vi "探头窗口-20.vi"() -> ()   [LabVIEW 2017]
panel:
  in  "更新数据":T1
  in  "停止信号":bool=TRUE
  out "更新数据？":bool=TRUE
  out "引用-切回列表模式？":refnum<vi>
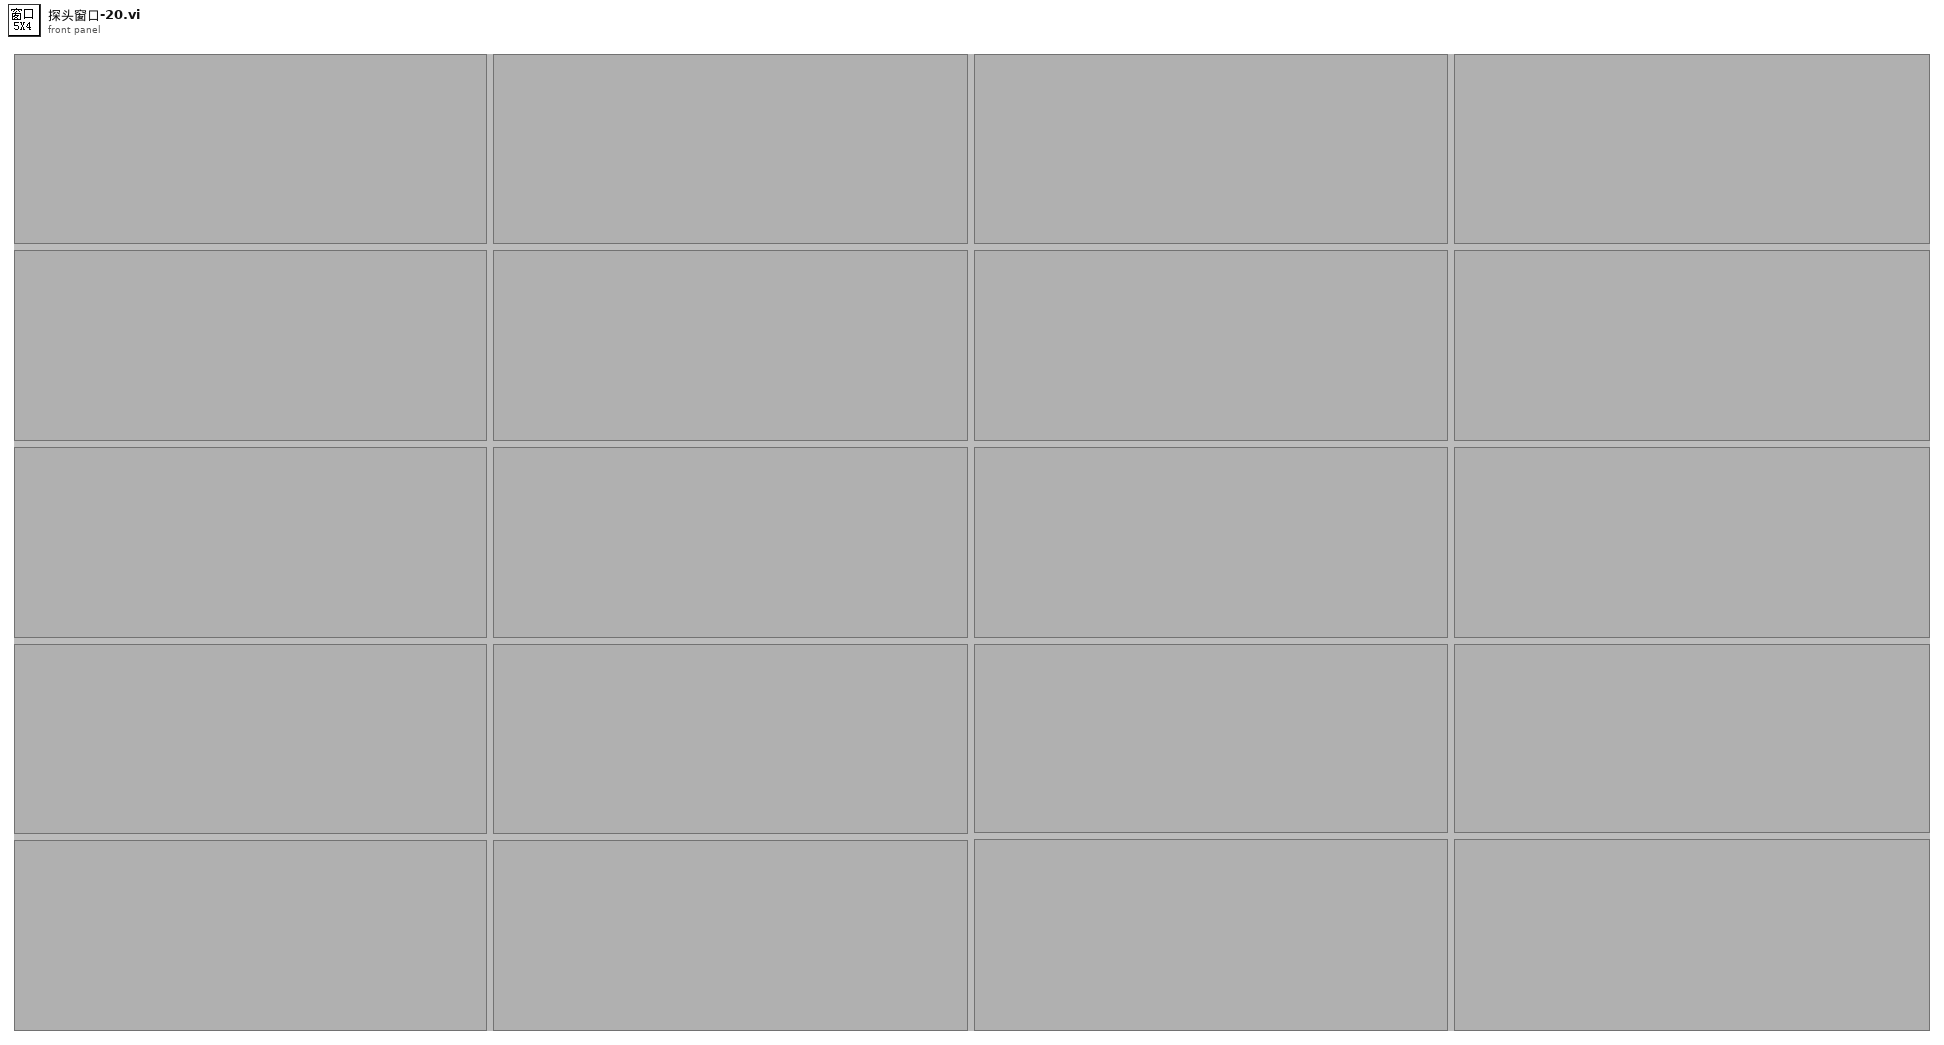
[diagram p1: front panel]
types:
  T1 = cluster{"探头启用状态？":bool[], "测量值":cluster{"X":timestamp, "Y":dbl}[], "限值":cluster{"限值1":dbl, "限值2":dbl, "探头限值":enum16{"一级限值", "二级限值"}}[], "报警状态":enum16{"正常", "一级报警", "二级报警", "累积报警"}[], "探头信息":string[], "累积剂量":cluster{"设备名称":string, "启用累积？":bool, "起始时间":timestamp, "累积剂量":dbl, "累积报警阈值":dbl}[]}
  T2 = cluster{"启用状态？":bool, "测量值":cluster{"X":timestamp, "Y":dbl}, "限值簇":cluster{"限值1":dbl, "限值2":dbl, "探头限值":enum16{"一级限值", "二级限值"}}, "报警状态":enum16{"正常", "一级报警", "二级报警", "累积报警"}, "探头信息":string, "探头地址":i32, "累积剂量":cluster{"设备名称":string, "启用累积？":bool, "起始时间":timestamp, "累积剂量":dbl, "累积报警阈值":dbl}}
  T3 = typedef "eventvkey.ctl" = enum16{"ASCII", "Enter", "Return", "Shift", "Ctrl", "Alt", "Cmd", "Opt", "Caps", "NumLock", "Clear", "Break", "Up", "Down", "Left", "Right", "Insert", "Delete", "Home", "End", "PageUp", "PageDown", "Escape", "Help", "Pause", "ScrollLock", "F1", "F2", "F3", "F4", "F5", "F6", "F7", "F8", "F9", "F10", "F11", "F12", "F13", "F14", "F15", "F16", "F17", "F18", "F19", "F20", "F21", "F22", "F23", "F24", "Play", "VolumeUp", "VolumeDown", "Mute", "Two Byte Char"}
  T4 = cluster{"限值1":dbl, "限值2":dbl, "探头限值":enum16{"一级限值", "二级限值"}}
  T5 = cluster{"限值1":dbl, "限值2":dbl, "探头限值":enum16{"一级限值", "二级限值"}}[]
  T6 = cluster{"设备名称":string, "启用累积？":bool, "起始时间":timestamp, "累积剂量":dbl, "累积报警阈值":dbl}[]
  T7 = cluster{"设备名称":string, "启用累积？":bool, "起始时间":timestamp, "累积剂量":dbl, "累积报警阈值":dbl}
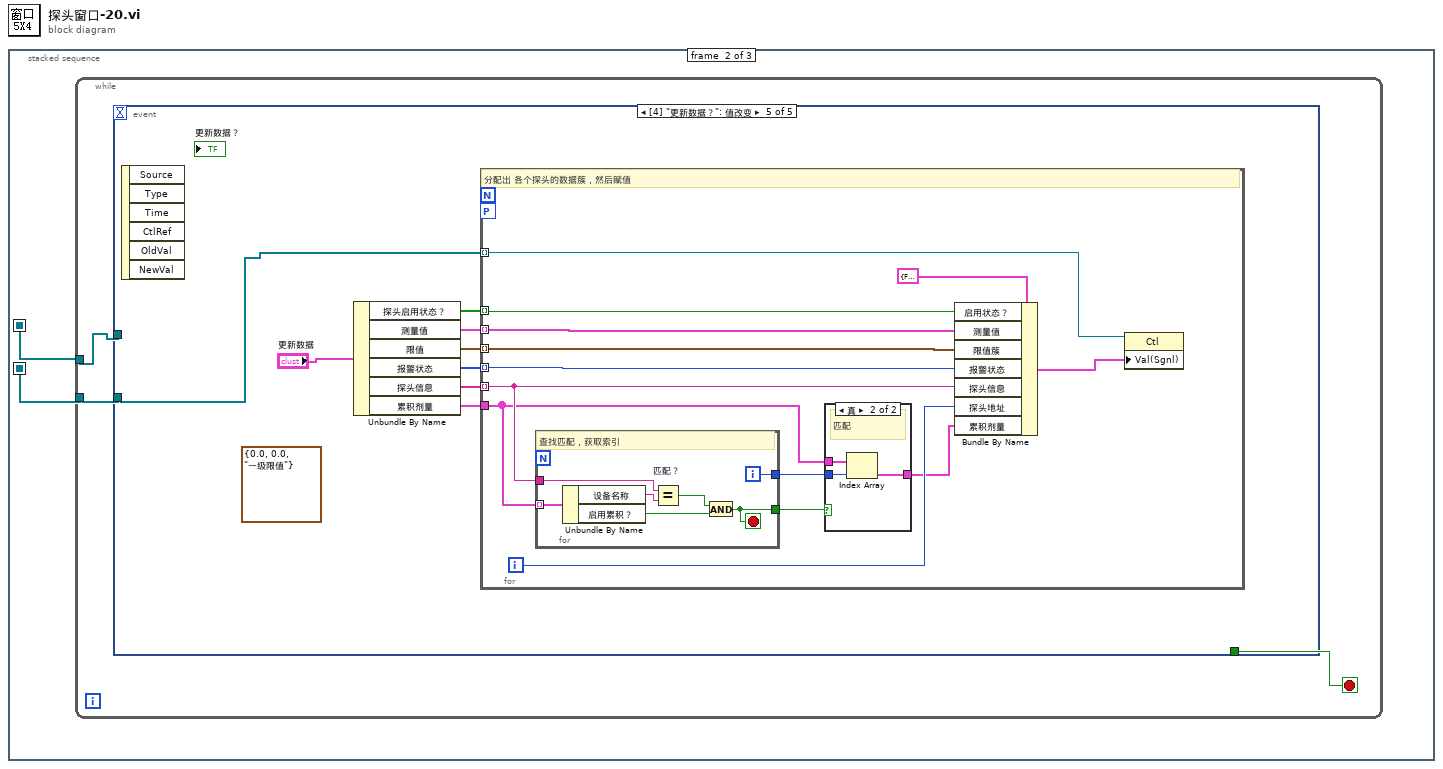
[diagram p0: block diagram]
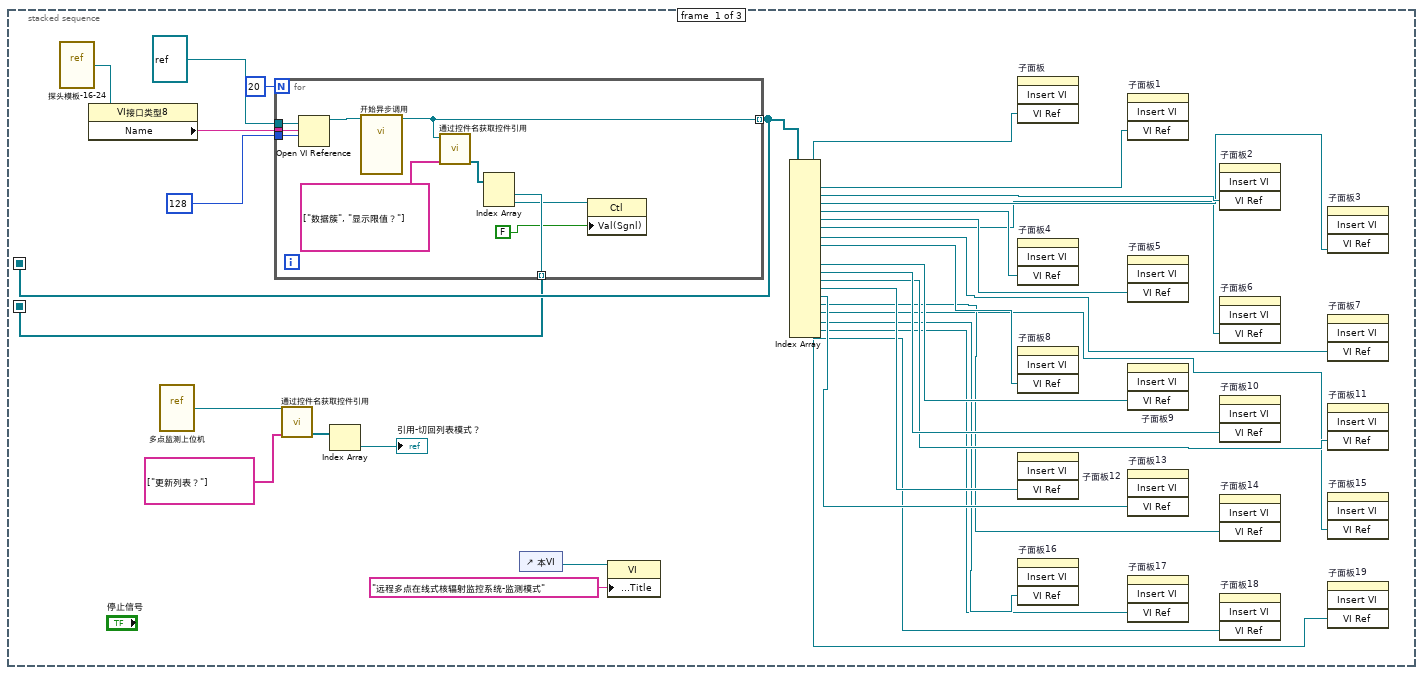
[diagram p2: hidden frame]
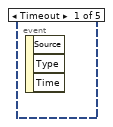
[diagram p3: hidden frame]
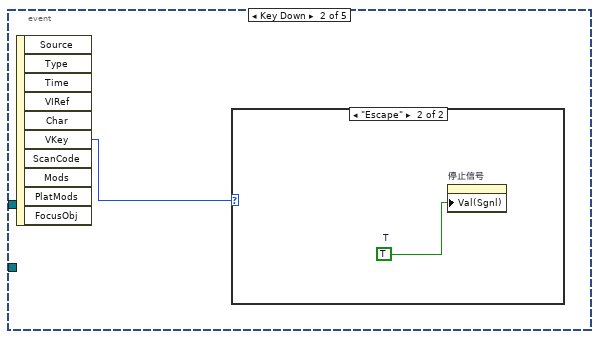
[diagram p4: hidden frame]
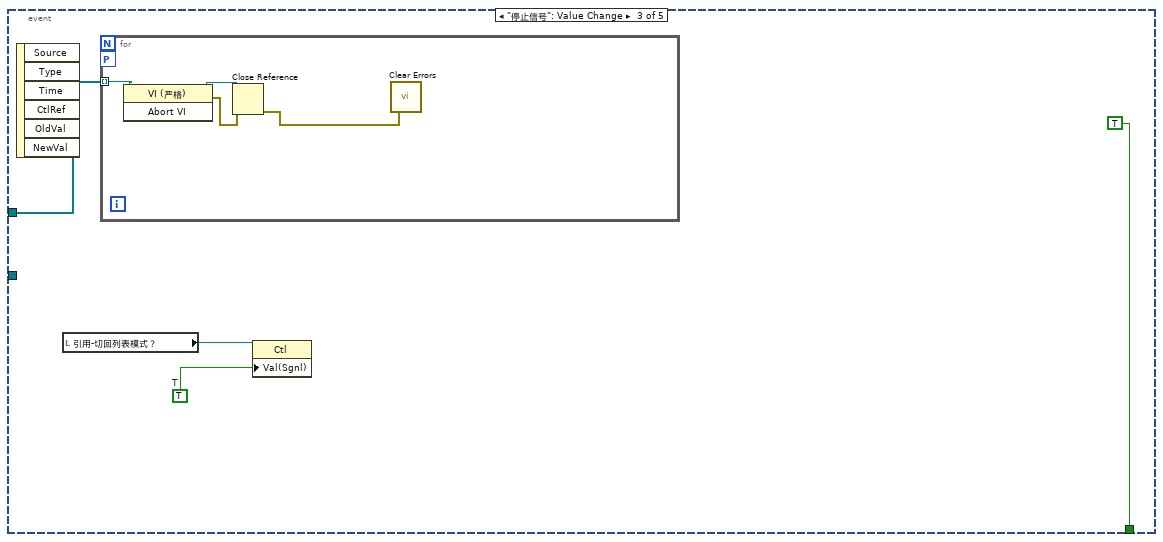
[diagram p6: hidden frame]
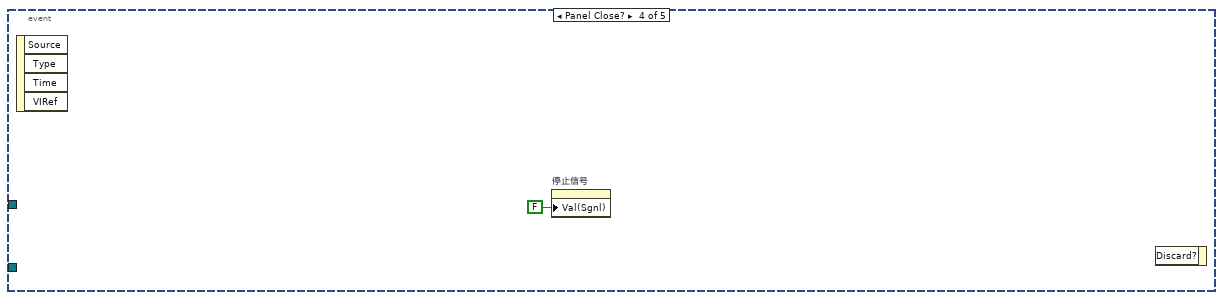
[diagram p7: hidden frame]
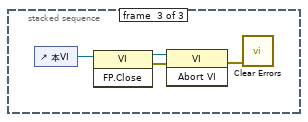
[diagram p9: hidden frame]
diagram:
  n1 = stacked-sequence {
    seq-local: [w28 _ _] -> [_ w45 _]
    seq-local: [w7 _ _] -> [_ w44 _]
    frame #0 {
      n2 = vi-ref "探头模板-16-24.vi"() -> (w33:refnum<vi>)
      n3 = property class="VI接口类型8"(reference=w33) -> ("Name"=w32:string)  [unwired: 1 in, 2 out]
      n4 = vi-ref "多点监测上位机.vi"() -> (w3:refnum<vi>)
      n5 = for {
        N: 20 -> [_]
        tunnel: w32 -> [w43]
        tunnel: 128 ("选项") -> [w42]
        tunnel: refnum<vi> refnum ("类型说明符VI引用句柄（仅用于类型）") -> [w41]
        tunnel: [w36] -> w28 mode=indexing
        tunnel: [w37] -> w7 mode=indexing
        n6 = Open VI Reference(type specifier VI Refnum (for type only)=w41, vi path=w43, options=w42) -> (vi reference=w38:refnum<vi>)  [unwired: 3 in, 1 out]
        n7 = call-by-ref "开始异步调用"(reference=w38) -> (reference out=w36:refnum<vi>)  [unwired: 13 in, 1 out]
        n8 = call "通过控件名获取控件引用.vi"("控件名数组"=string[] ["数据簇", "显示限值？"], "VI引用"=w36) -> ("控件引用输出"=w40:refnum<vi>[])  [unwired: 7 in, 2 out]
        n9 = Index Array(array=w40) -> (element #1=w37:refnum<vi>, element #2=w35:refnum<vi>)  [unwired: 2 in]
        n10 = property class="Ctl"(reference=w35, "Val(Sgnl)"=FALSE) -> ()  [unwired: 1 in, 2 out]
      }
      n11 = call "通过控件名获取控件引用.vi"("控件名数组"=string[] ["更新列表？"], "VI引用"=w3) -> ("控件引用输出"=w5:refnum<vi>[])  [unwired: 7 in, 2 out]
      n12 = Index Array(array=w5) -> (element=→"引用-切回列表模式？":refnum<vi>)  [unwired: 1 in]
      n13 = control-ref of="本VI"() -> (w2:refnum<vi>)
      n14 = property class="VI"(reference=w2, "Front Panel.Title"="远程多点在线式核辐射监控系统-监测模式" ("前面板窗口:标题")) -> ()  [unwired: 1 in, 2 out]
      n15 = Index Array(array=w28) -> (element #1=w27:refnum<vi>, element #2=w26:refnum<vi>, element #3=w25:refnum<vi>, element #4=w24:refnum<vi>, element #5=w23:refnum<vi>, element #6=w22:refnum<vi>, element #7=w21:refnum<vi>, element #8=w20:refnum<vi>, element #9=w19:refnum<vi>, element #10=w18:refnum<vi>, element #11=w17:refnum<vi>, element #12=w16:refnum<vi>, element #13=w15:refnum<vi>, element #14=w14:refnum<vi>, element #15=w13:refnum<vi>, element #16=w12:refnum<vi>, element #17=w11:refnum<vi>, element #18=w10:refnum<vi>, element #19=w9:refnum<vi>, element #20=w8:refnum<vi>)  [unwired: 20 in]
      n16 = invoke on="子面板" class="子面板" method="Insert VI"("VI Ref"=w27) -> ()  [unwired: 3 in, 4 out]
      n17 = invoke on="子面板4" class="SubPnl" method="Insert VI"("VI Ref"=w23) -> ()  [unwired: 3 in, 4 out]
      n18 = invoke on="子面板8" class="SubPnl" method="Insert VI"("VI Ref"=w19) -> ()  [unwired: 3 in, 4 out]
      n19 = invoke on="子面板12" class="SubPnl" method="Insert VI"("VI Ref"=w15) -> ()  [unwired: 3 in, 4 out]
      n20 = invoke on="子面板16" class="SubPnl" method="Insert VI"("VI Ref"=w11) -> ()  [unwired: 3 in, 4 out]
      n21 = invoke on="子面板1" class="SubPnl" method="Insert VI"("VI Ref"=w26) -> ()  [unwired: 3 in, 4 out]
      n22 = invoke on="子面板5" class="SubPnl" method="Insert VI"("VI Ref"=w22) -> ()  [unwired: 3 in, 4 out]
      n23 = invoke on="子面板9" class="SubPnl" method="Insert VI"("VI Ref"=w18) -> ()  [unwired: 3 in, 4 out]
      n24 = invoke on="子面板13" class="SubPnl" method="Insert VI"("VI Ref"=w14) -> ()  [unwired: 3 in, 4 out]
      n25 = invoke on="子面板17" class="SubPnl" method="Insert VI"("VI Ref"=w10) -> ()  [unwired: 3 in, 4 out]
      n26 = invoke on="子面板2" class="SubPnl" method="Insert VI"("VI Ref"=w25) -> ()  [unwired: 3 in, 4 out]
      n27 = invoke on="子面板6" class="SubPnl" method="Insert VI"("VI Ref"=w21) -> ()  [unwired: 3 in, 4 out]
      n28 = invoke on="子面板10" class="SubPnl" method="Insert VI"("VI Ref"=w17) -> ()  [unwired: 3 in, 4 out]
      n29 = invoke on="子面板14" class="SubPnl" method="Insert VI"("VI Ref"=w13) -> ()  [unwired: 3 in, 4 out]
      n30 = invoke on="子面板18" class="SubPnl" method="Insert VI"("VI Ref"=w9) -> ()  [unwired: 3 in, 4 out]
      n31 = invoke on="子面板3" class="SubPnl" method="Insert VI"("VI Ref"=w24) -> ()  [unwired: 3 in, 4 out]
      n32 = invoke on="子面板7" class="SubPnl" method="Insert VI"("VI Ref"=w20) -> ()  [unwired: 3 in, 4 out]
      n33 = invoke on="子面板11" class="SubPnl" method="Insert VI"("VI Ref"=w16) -> ()  [unwired: 3 in, 4 out]
      n34 = invoke on="子面板15" class="SubPnl" method="Insert VI"("VI Ref"=w12) -> ()  [unwired: 3 in, 4 out]
      n35 = invoke on="子面板19" class="SubPnl" method="Insert VI"("VI Ref"=w8) -> ()  [unwired: 3 in, 4 out]
    }
    frame #1 {
      n36 = while {
        tunnel: w45 -> [w47]
        tunnel: w44 -> [w46]
        stop <- w48 stop-if-true
        n37 = event shown="[4] \"更新数据？\": 值改变" {
          selector: _ -> [_ _ _ _ _]
          dyn-events: _ -> [_ _ _ _ _]
          timeout: _ -> [_ _ _ _ _]
          tunnel: [_ _ TRUE ("放弃？") _ _] -> w48
          tunnel: w47 -> [_ _ w53 _ _]
          tunnel: w46 -> [_ _ _ _ w60]
          event Timeout {
            n38 = event-data() -> ()  [unwired: 1 in, 3 out]
          }
          event Key Down {
            n39 = event-data() -> ("VKey"=w49:T3)  [unwired: 1 in, 9 out]
            n40 = case shown="\"Escape\"" w49 {
              frame "ASCII", Default {
              }
              frame "Escape" {
                w50 = TRUE  # T
                n41 = property on="停止信号" class="Bool (严格)"("Val(Sgnl)"=w50) -> ()  [unwired: 2 in, 2 out]
              }
            }
          }
          event "停止信号": Value Change {
            w52 = TRUE  # T
            n42 = event-data() -> ()  [unwired: 1 in, 6 out]
            n43 = local read "引用-切回列表模式？"() -> (w51:refnum<vi>)
            n44 = for {
              tunnel: w53 -> [w58] mode=indexing
              workers-P: _ -> [_]
              n45 = invoke class="VI (严格)" method="Abort VI"(reference=w58) -> (reference out=w56:refnum<vi>, error out=w57:errorcluster)  [unwired: 2 in, 1 out]
              n46 = Close Reference(reference=w56, error in (no error)=w57) -> (error out=w55:errorcluster)
              n47 = call <vilib>:"Clear Errors.vi"("error in (no error)"=w55) -> ()  [unwired: 5 in, 2 out]
            }
            n48 = property class="Ctl"(reference=w51, "Val(Sgnl)"=w52) -> ()  [unwired: 1 in, 2 out]
          }
          event Panel Close? {
            n49 = event-data() -> ()  [unwired: 1 in, 4 out]
            n50 = property on="停止信号" class="Bool (严格)"("Val(Sgnl)"=FALSE ("值(信号)")) -> ()  [unwired: 2 in, 2 out]
            n51 = event-data() -> ()  [unwired: 2 in, 1 out]
          }
          event "更新数据？": Value Change {
            (unwired) T4 {"限值1"=0.0, "限值2"=0.0, "探头限值"=enum."一级限值"} ("探头限值簇")
            n52 = event-data() -> ()  [unwired: 1 in, 6 out]
            n53 = Unbundle By Name("更新数据") -> ("探头启用状态？"=w61:bool[], "测量值"=w62:cluster{"X":timestamp, "Y":dbl}[], "限值"=w63:T5, "报警状态"=w64:enum16{"正常", "一级报警", "二级报警", "累积报警"}[], "探头信息"=w65:string[], "累积剂量"=w66:T6)
            n54 = for {
              tunnel: w61 -> [w80] mode=indexing
              tunnel: w62 -> [w79] mode=indexing
              tunnel: w63 -> [w78] mode=indexing
              tunnel: w64 -> [w77] mode=indexing
              tunnel: w65 -> [w72] mode=indexing
              workers-P: _ -> [_]
              tunnel: w60 -> [w75] mode=indexing
              tunnel: w66 -> [w71]
              i -> [w73]
              # "分配出 各个探头的数据簇，然后赋值"
              n55 = for {
                tunnel: w71 -> [w90] mode=indexing
                tunnel: w72 -> [w88]
                tunnel: [w85] -> w70
                tunnel: [w84] -> w69
                i -> [w85]
                stop <- w84 stop-if-true
                # "查找匹配，获取索引"
                n56 = Unbundle By Name(w90) -> ("设备名称"=w89:string, "启用累积？"=w86:bool)
                n57 = Equal? "匹配？"(x=w88, y=w89) -> (x = y?=w87:bool)
                n58 = And(x=w87, y=w86) -> (x .and. y?=w84:bool)
              }
              n59 = case shown="真" w69 {
                tunnel: w71 -> [_ w83]
                tunnel: w70 -> [_ w82]
                tunnel: [_ w81] -> w68
                frame False {
                  # "不匹配"
                }
                frame True {
                  # "匹配"
                  n60 = Index Array(array=w83, index=w82) -> (element=w81:T7)
                }
              }
              n61 = Bundle By Name(cluster=T2 {"启用状态？"=FALSE, "测量值"={"X"=timestamp(0 s since 1904-01-01), "Y"=0.0}, "限值簇"={"限值1"=0.0, "限值2"=0.0, "探头限值"=enum."一级限值"}, "报警状态"=enum."正常", "探头信息"="", "探头地址"=0, "累积剂量"={"设备名称"="", "启用累积？"=FALSE, "起始时间"=timestamp(0 s since 1904-01-01), "累积剂量"=0.0, "累积报警阈值"=0.0}} ("输出簇"), "启用状态？"=w80, "测量值"=w79, "限值簇"=w78, "报警状态"=w77, "探头信息"=w72, "探头地址"=w73, "累积剂量"=w68) -> (w74:T2)
              n62 = property class="Ctl"(reference=w75, "Val(Sgnl)"=w74) -> ()  [unwired: 1 in, 2 out]
            }
          }
        }
      }
    }
    frame #2 {
      n63 = control-ref of="本VI"() -> (w94:refnum<vi>)
      n64 = invoke class="VI" method="FP.Close"(reference=w94) -> (reference out=w93:refnum<vi>, error out=w92:errorcluster)  [unwired: 2 in, 1 out]
      n65 = invoke class="VI" method="Abort VI"(reference=w93, error in=w92) -> (error out=w91:errorcluster)  [unwired: 1 in, 2 out]
      n66 = call <vilib>:"Clear Errors.vi"("error in (no error)"=w91) -> ()  [unwired: 5 in, 2 out]
    }
  }
